vi "Gray Out Enable.vi"(6 "Controls[]":refnum<vi>[](array[refnum]), 7 "Disabled":T1(ring), 8 "Error In":errorcluster) -> (0 "Error Out":errorcluster)   [LabVIEW 2014]
doc: "This VI grayes out controls or make them enable"
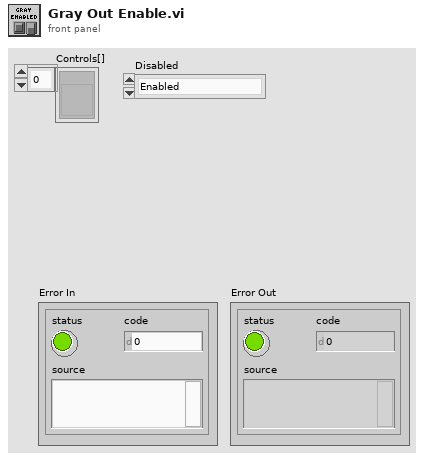
[diagram p1: front panel]
types:
  T1 = enum8{"Enabled", "Disabled", "Disabled and Grayed Out"}
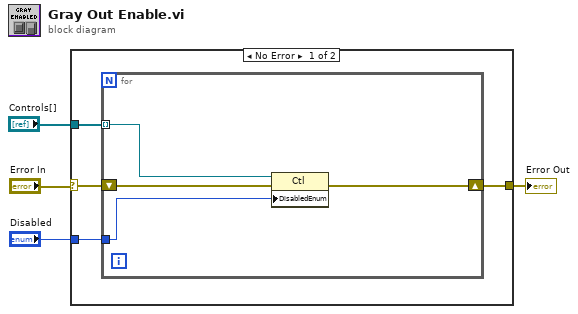
[diagram p0: block diagram]
diagram:
  n1 = case shown="No Error" "Error In" {
    selector: "Error In" -> [w7 w13]
    tunnel: "Controls[]" -> [w8 _]
    tunnel: [w6 w13] -> w2
    tunnel: "Disabled" -> [w5 _]
    frame No Error {
      n2 = for {
        tunnel: w8 -> [w11] mode=indexing
        shift-right: [w10] -> w6
        shift-left: w7 -> [w12]
        tunnel: w5 -> [w9]
        n3 = property class="Ctl"(reference=w11, error in=w12, "DisabledEnum"=w9) -> (error out=w10:errorcluster)  [unwired: 1 out]
      }
    }
    frame Error {
    }
  }
  "Error Out" <- w2
